vi "SelectSlidewithMouseUp.vi"(2 "SlideInfo":T2[](array[typedef]), 3 "Mouse":T1) -> (0 "index":i32, 1 "Slide":T2)   [LabVIEW 2014]
uses:
  SlideTypeDef.ctl
  <vilib>/Utility/miscctls.llb/LVMouseTypeDef.ctl
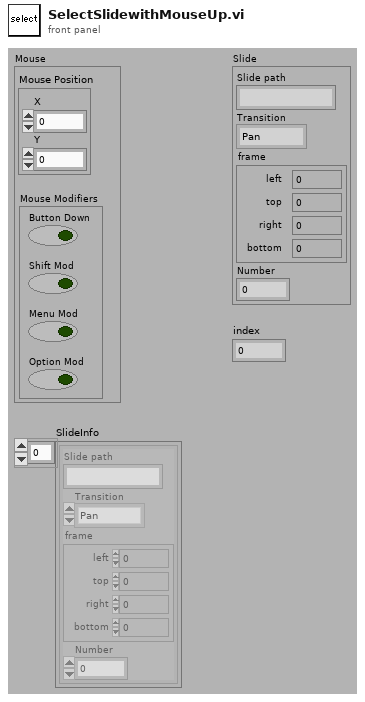
[diagram p1: front panel]
types:
  T1 = typedef "LVMouseTypeDef.ctl" = cluster{"Mouse Position":cluster{"X":i32, "Y":i32}, "Mouse Modifiers":cluster{"Button Down":bool, "Shift Mod":bool, "Menu Mod":bool, "Option Mod":bool}}
  T2 = typedef "SlideTypeDef.ctl" = cluster{"Slide path":string, "Transition":enum16{"Pan", "Zoom-pan-zoom", "Zoom-wait-Zoom"}, "frame":cluster{"left":i16, "top":i16, "right":i16, "bottom":i16}, "Number":i32}
  T3 = cluster{"left":i16, "top":i16, "right":i16, "bottom":i16}
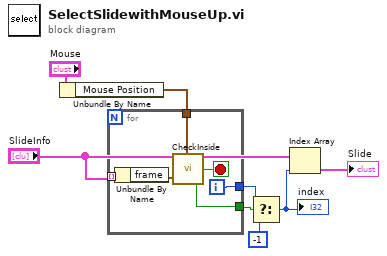
[diagram p0: block diagram]
diagram:
  n1 = Unbundle By Name("Mouse") -> ("Mouse Position"=w1:cluster{"X":i32, "Y":i32})
  n2 = for {
    tunnel: "SlideInfo" -> [w13] mode=indexing
    tunnel: w1 -> [w12]
    tunnel: [w11] -> w4
    tunnel: [w10] -> w5
    i -> [w11]
    stop <- w10 stop-if-true
    n3 = Unbundle By Name(w13) -> ("frame"=w9:T3)
    n4 = call "CheckInside.vi"("rect"=w9, "Coords"=w12) -> ("Inside?"=w10:bool)
  }
  n5 = Select(t=w4, s=w5, f=-1) -> (s? t:f=w6:i32)
  "index" <- w6
  n6 = Index Array(array="SlideInfo", index=w6) -> (element=→"Slide":T2)
